vi "read sorted dictionary.vi"(8 "error in":errorcluster, 11 "data dictionary in":refnum<class "data dictionary.lvclass">) -> (0 "error out":errorcluster, 1 "tags by type":cluster{"indices":i32[], "names":string[]}[](array[cluster]), 2 "types":T1[](array[typedef]), 3 "data dictionary out":refnum<class "data dictionary.lvclass">)   [LabVIEW 2013, in "tag bus.lvlib" / "data dictionary.lvclass"]
doc: "Reads the entire data dictionary and returns it as a sorted set of tag names, organized by data type. This is very inefficient, duplicating the entire tag list and performing a sorting algorithm on this list."
uses:
  data dictionary.lvclass
  tag/Data Type.ctl
  data dictionary.lvclass/data dictionary.ctl
  tag/tag descriptor.lvclass
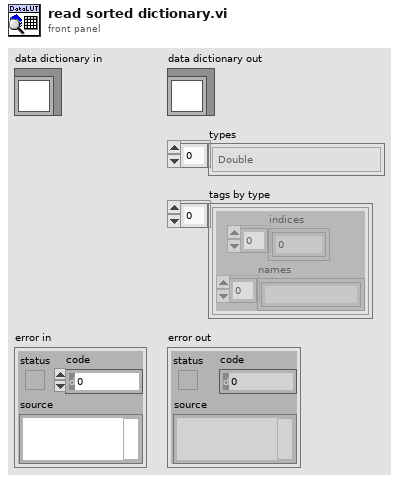
[diagram p1: front panel]
types:
  T1 = typedef "tag bus.lvlib/tag descriptor.lvclass/Data Type.ctl" = enum16{"Double", "Single", "I64", "I32", "I16", "I8", "U64", "U32", "U16", "U8", "Boolean", "String", "Array of Double", "Array of Single", "Array of I64", "Array of I32", "Array of I16", "Array of I8", "Array of U64", "Array of U32", "Array of U16", "Array of U8", "Array of Boolean", "Array of String"}
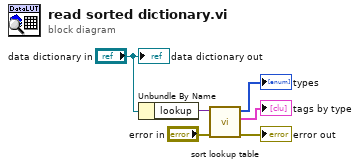
[diagram p0: block diagram]
diagram:
  n1 = Unbundle By Name("data dictionary in") -> ("lookup"=w3:variant)
  n2 = call "sort lookup table.vi"("error in (no error)"="error in", "lookup"=w3) -> ("error out"=→"error out":errorcluster, "tags by type"=→"tags by type":cluster{"indices":i32[], "names":string[]}[], "types"=→"types":T1[])  [unwired: 7 in]
  "data dictionary out" <- "data dictionary in"
